vi "read field from DSC.vi"() -> (6 "Bx, By, Bz":dbl[](array[numeric]), 7 "error out":errorcluster)   [LabVIEW 2013]
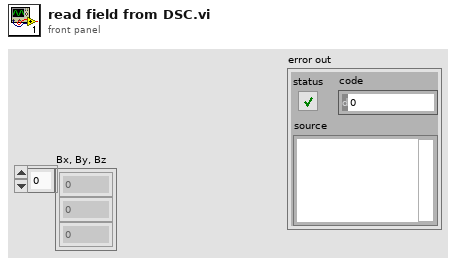
[diagram p1: front panel]
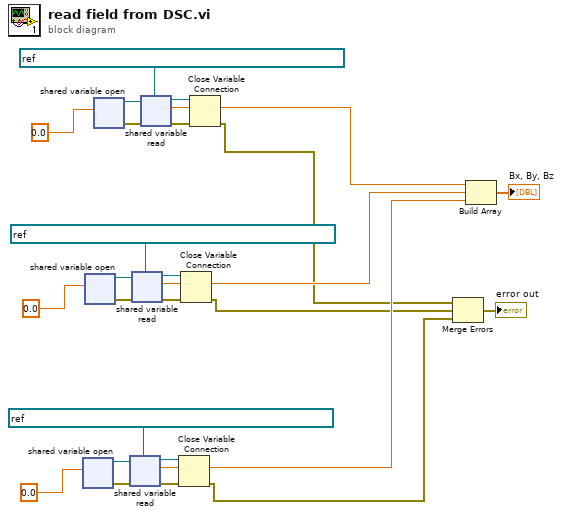
[diagram p0: block diagram]
diagram:
  n1 = shared-variable-open(refnum<k21> "ni.var.psp://housesoftheholy/Leiden CF900/CF Output Z" ("shared variable refnum in"), 0.0) -> (w11:refnum<k21>, w13:errorcluster)  [unwired: 2 in]
  n2 = shared-variable-open(refnum<k21> "ni.var.psp://housesoftheholy/Leiden CF900/CF Output Y" ("shared variable refnum in"), 0.0) -> (w18:refnum<k21>, w16:errorcluster)  [unwired: 2 in]
  n3 = shared-variable-open(refnum<k21> "ni.var.psp://housesoftheholy/Leiden CF900/CF Output X" ("shared variable refnum in"), 0.0) -> (w23:refnum<k21>, w25:errorcluster)  [unwired: 2 in]
  n4 = shared-variable-read(w11, w13) -> (w12:refnum<k21>, w14:errorcluster, w6:dbl)  [unwired: 1 out]
  n5 = shared-variable-read(w18, w16) -> (w17:refnum<k21>, w15:errorcluster, w7:dbl)  [unwired: 1 out]
  n6 = shared-variable-read(w23, w25) -> (w24:refnum<k21>, w26:errorcluster, w8:dbl)  [unwired: 1 out]
  n7 = Close Variable Connection(8:w14, 11:w12) -> (0:w2:errorcluster)
  n8 = Close Variable Connection(8:w15, 11:w17) -> (0:w3:errorcluster)
  n9 = Close Variable Connection(8:w26, 11:w24) -> (0:w4:errorcluster)
  n10 = Merge Errors(w4, w3, w2) -> (→"error out":errorcluster)
  n11 = Build Array(w8, w7, w6) -> (→"Bx, By, Bz":dbl[])
